vi "callpb_photo.vi"() -> ()   [LabVIEW 2018]
uses:
  <vilib>/addons/VIRobotics/opencv_yiku/ctls/scalar3.ctl
  <vilib>/addons/VIRobotics/opencv_yiku/Mat/Mat_8U/Mat_8U.lvclass
  C:/Program Files/National Instruments/LabVIEW 2018_64bit/vi.lib/addons/VIRobotics/opencv_yiku/Mat/Mat/Mat.lvclass
  <vilib>/addons/VIRobotics/opencv_yiku/Mat/Mat_32F/Mat_32F.lvclass
  <vilib>/addons/VIRobotics/opencv_yiku/Mat/Create_Mat_32F.vi
  <vilib>/addons/VIRobotics/opencv_yiku/Mat/Mat/Mat_release.vi
  <vilib>/addons/VIRobotics/opencv_yiku/Mat/Mat/Mat_length.vi
  <vilib>/Utility/file.llb/Read Delimited Spreadsheet (string).vi
  <vilib>/addons/VIRobotics/opencv_yiku/opencv_yiku.lvlib
  <vilib>/addons/VIRobotics/opencv_yiku/dnn/Net/Net.lvclass
  <vilib>/addons/VIRobotics/opencv_yiku/Mat/Mat/Mat.lvclass
panel:
  out "label":string
  out "picture":picture
  out "大小":i32[](array[numeric])
  out "max index(es)":i32
  out "max value":sgl format="%#_13g"
  out "最终结果":sgl[](array[numeric])
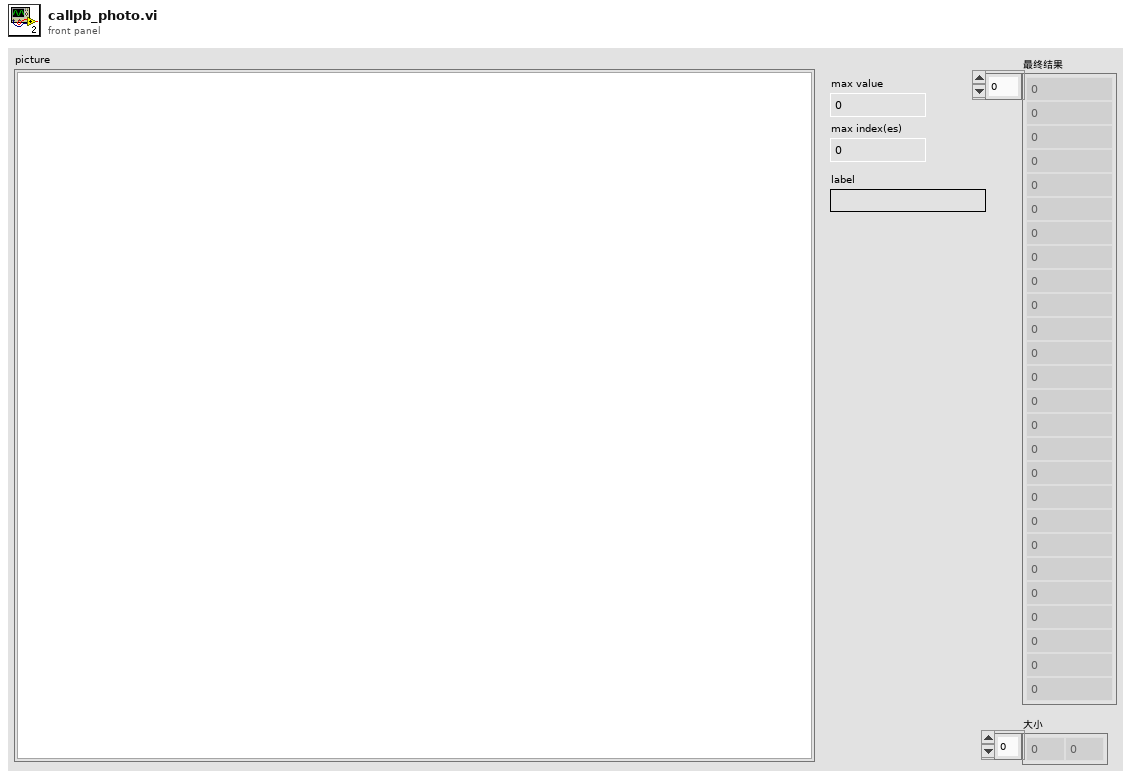
[diagram p1: front panel]
types:
  T1 = typedef "opencv_yiku.lvlib/scalar3.ctl" = cluster{"x":dbl, "y":dbl, "z":dbl}
  T2 = enum16{"COLOR_BGR2BGRA", "COLOR_BGRA2BGR", "COLOR_BGR2RGBA", "COLOR_RGBA2BGR", "COLOR_BGR2RGB", "COLOR_BGRA2RGBA", "COLOR_BGR2GRAY", "COLOR_RGB2GRAY", "COLOR_GRAY2BGR", "COLOR_GRAY2BGRA"}
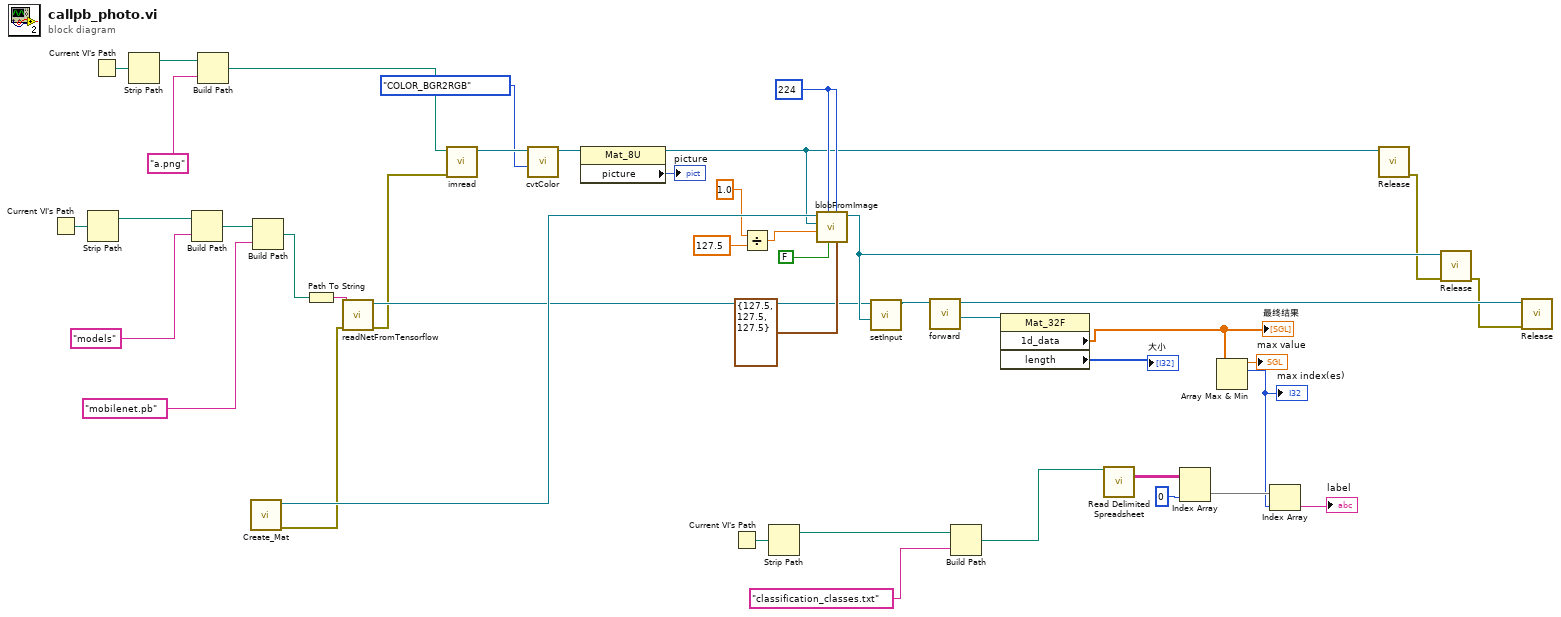
[diagram p0: block diagram]
diagram:
  w31 = 224 ("rows")
  n1 = Current VI's Path() -> (path=w38:path)
  n2 = Strip Path(path=w38) -> (stripped path=w35:path)  [unwired: 1 out]
  n3 = Current VI's Path() -> (path=w10:path)
  n4 = Strip Path(path=w10) -> (stripped path=w9:path)  [unwired: 1 out]
  n5 = Build Path(base path=w35, name or relative path="models") -> (appended path=w33:path)
  n6 = Build Path(base path=w9, name or relative path="a.png") -> (appended path=w8:path)
  n7 = call-poly <vilib>:"Create_Mat.vi"() -> ("error out"=w19:errorcluster, "Mat_32F_out"=w43:refnum<class "Mat_32F.lvclass">)  [unwired: 10 in]
  n8 = Build Path(base path=w33, name or relative path="mobilenet.pb") -> (appended path=w36:path)
  n9 = Path To String(path=w36) -> (string=w44:string)
  n10 = call <vilib>:"readNetFromTensorflow.vi"("error in (no error)"=w19, "pbfile"=w44) -> ("error out"=w5:errorcluster, "Net out"=w6:refnum<class "Net.lvclass">)  [unwired: 8 in]
  n11 = call <vilib>:"imread.vi"("error in (no error)"=w5, "path"=w8) -> ("Mat out"=w21:refnum<class "Mat_8U.lvclass">)  [unwired: 8 in, 1 out]
  n12 = call <vilib>:"cvtColor.vi"("dstCn"=T2."COLOR_BGR2RGB", "src"=w21) -> ("src out"=w18:refnum<class "Mat_8U.lvclass">)  [unwired: 7 in, 2 out]
  n13 = property class="Mat_8U"(reference=w18) -> (reference out=w16:refnum<class "Mat_8U.lvclass">, "picture"=→"picture":picture)  [unwired: 1 in, 1 out]
  n14 = Current VI's Path() -> (path=w4:path)
  n15 = Divide(x=1.0 ("k"), y=127.5) -> (x/y=w25:dbl)
  n16 = Strip Path(path=w4) -> (stripped path=w3:path)  [unwired: 1 out]
  n17 = call <vilib>:"blobFromImage.vi"("mean"=T1 {"x"=127.5, "y"=127.5, "z"=127.5}, "rows"=w31, "swapRB"=FALSE, "columns"=w31, "scale"=w25, "Mat in"=w16, "dst"=w43) -> ("dst out"=w42:refnum<class "Mat_32F.lvclass">)  [unwired: 3 in, 1 out]
  n18 = call <vilib>:"setInput.vi"("Mat"=w42, "Net in"=w6) -> ("Net out"=w30:refnum<class "Net.lvclass">)  [unwired: 8 in, 1 out]
  n19 = call <vilib>:"forward.vi"("Net in"=w30) -> ("Mat out"=w29:refnum<class "Mat_32F.lvclass">, "Net out"=w41:refnum<class "Net.lvclass">)  [unwired: 8 in, 1 out]
  n20 = Build Path(base path=w3, name or relative path="classification_classes.txt") -> (appended path=w1:path)
  n21 = property class="Mat_32F"(reference=w29) -> ("1d_data"=w24:sgl[], "length"=→"大小":i32[])  [unwired: 1 in, 2 out]
  "最终结果" <- w24
  n22 = call-poly <vilib>:"Read Delimited Spreadsheet.vi"("file path (dialog if empty)"=w1) -> ("all rows"=w15:string[][])  [unwired: 9 in, 5 out]
  n23 = Index Array(array=w15, index (col)=0 ("disabled index (col)")) -> (element=w13:string[])  [unwired: 1 in]
  n24 = Array Max & Min(array=w24) -> (max value=→"max value":sgl, max index (indices)=w12:i32)  [unwired: 2 out]
  "max index(es)" <- w12
  n25 = Index Array(array=w13, index=w12) -> (element=→"label":string)
  n26 = call-poly <vilib>:"Release.vi"("Mat in"=w16) -> ("error out"=w40:errorcluster)  [unwired: 10 in]
  n27 = call-poly <vilib>:"Release.vi"("error in (no error)"=w40, "Mat in"=w42) -> ("error out"=w39:errorcluster)  [unwired: 9 in]
  n28 = call-poly <vilib>:"Release.vi"("error in (no error)"=w39, "Net in"=w41) -> ()  [unwired: 9 in, 1 out]
